vi "AbsoluteIMU-DM.vi"(0 "Operation":u8(ring) items=["Read Accl", "Read Compass", "Read Magnetic Field", "Read Accl & Compass", "Read Gyro", "Begin Compass Calib", "End Compass Calib", "Sens-2G", "Sens-4G", "Sens-8G", "Sens-16G"], 2 "NXT":T3={"Hardware"="NXT", "Flattened String"=""}, 3 "Input Port":T2=3 items=["Port 1", "Port 2", "Port 3", "Port 4"]) -> (1 "output cluster":T1={"X Tilt"=0, "Y Tilt"=0, "Z Tilt"=0, "X Accel"=0, "Y Accel"=0, "Z accel"=0, "X Gyro"=0, "Y Gyro"=0, "Z Gyro"=0, "X Mag"=0, "Y Mag"=0, "Z Mag"=0, "Heading"=0, "Success?"=TRUE}, 4 "NXT dup":T3 caption="NXT")   [LabVIEW 2011]
uses:
  <vilib>/NXT/Subs/LVHSConnector.ctl
  <vilib>/NXT/Block Support/NXT_InputPort.ctl
  <vilib>/NXT/Block Support/HWPage.SensorType.ctl
  <vilib>/NXT/Block Support/HWPage.SensorMode.ctl
panel:
  out "last Z Magnetic Field":i16
  out "last Y Magnetic Field":i16
  out "last X Magnetic Field":i16
  out "Heading":i16
  out "Z Accel":i16
  out "Y Accel":i16
  out "X Accel":i16
  out "Z Tilt":i16
  out "Y Tilt":i16
  out "X Tilt":i16
  out "last Z Gyro":i16
  out "last Y Gyro":i16
  out "last X Gyro":i16
  out "last X Tilt":i16
  out "last Y Tilt":i16
  out "last Z Tilt":i16
  out "last Y Accel":i16
  out "last X Accel":i16
  out "last Z Accel":i16
  out "last Heading":i16
  in  "Address":u8=34 format="%x"
  out "Boolean":bool=TRUE caption="Yes / No"
  out "Y Gyro":i16
  out "X Gyro":i16
  out "Z Gyro":i16
  out "Y Magnetic Field":i16
  out "X Magnetic Field":i16
  out "Z Magnetic Field":i16
  # "mindsensors.com\nCopyright (c) 2013 by mindsensors.com\nEmail: info (<at>) mindsensors (<dot>) com\n\nThis program is free software. You can redistribute it and/or modify\nit under the terms of the GNU General Public License as published by\nthe Free Software Foundation; version 3 of the License.\nRead the license at: http://www.gnu.org/licenses/gpl.txt"
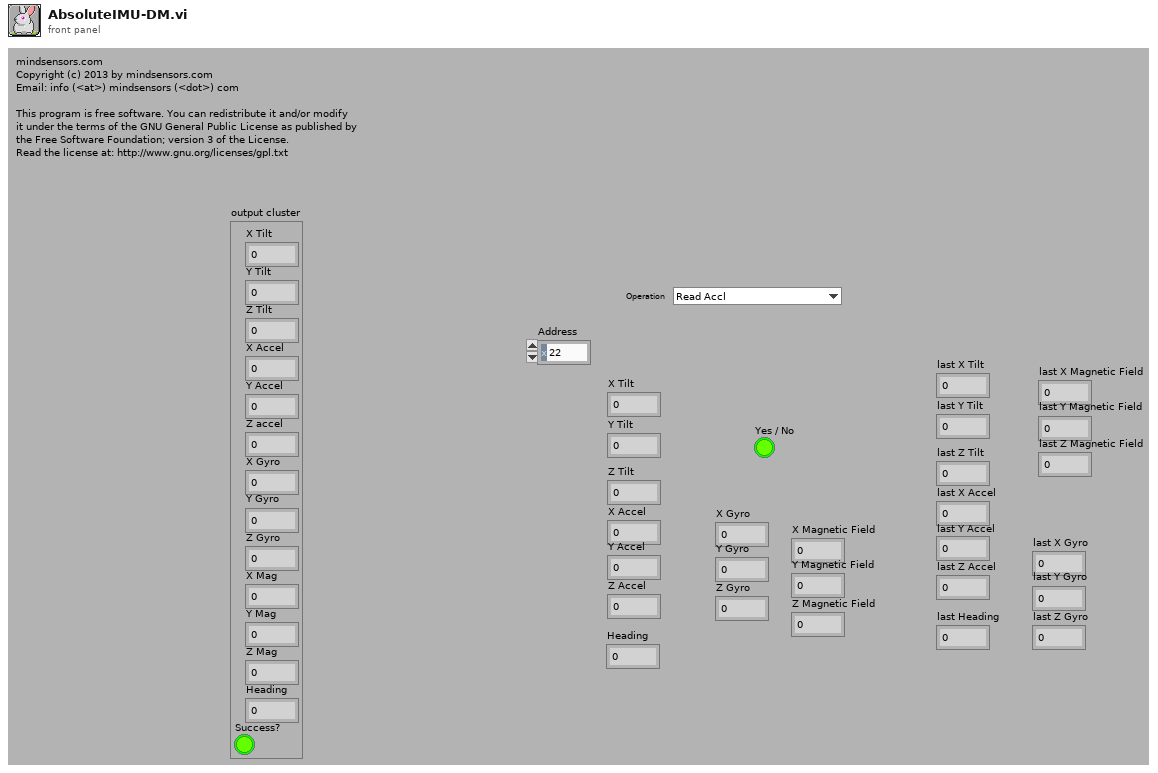
[diagram p1: front panel]
types:
  T1 = cluster{"X Tilt":i32, "Y Tilt":i32, "Z Tilt":i32, "X Accel":i32, "Y Accel":i32, "Z accel":i32, "X Gyro":i32, "Y Gyro":i32, "Z Gyro":i32, "X Mag":i32, "Y Mag":i32, "Z Mag":i32, "Heading":i32, "Success?":bool}
  T2 = typedef "NXT_InputPort.ctl" = u8
  T3 = typedef "LVHSConnector.ctl" = cluster{"Hardware":string, "Flattened String":string}
  T4 = typedef "HWPage.SensorType.ctl" = u8
  T5 = typedef "HWPage.SensorMode.ctl" = u8
  T6 = cluster{i16, i16, i16, i16, i16, i16, i16, i16, i16, i16, i16, i16, "last X Tilt":i32, "Success?":bool}
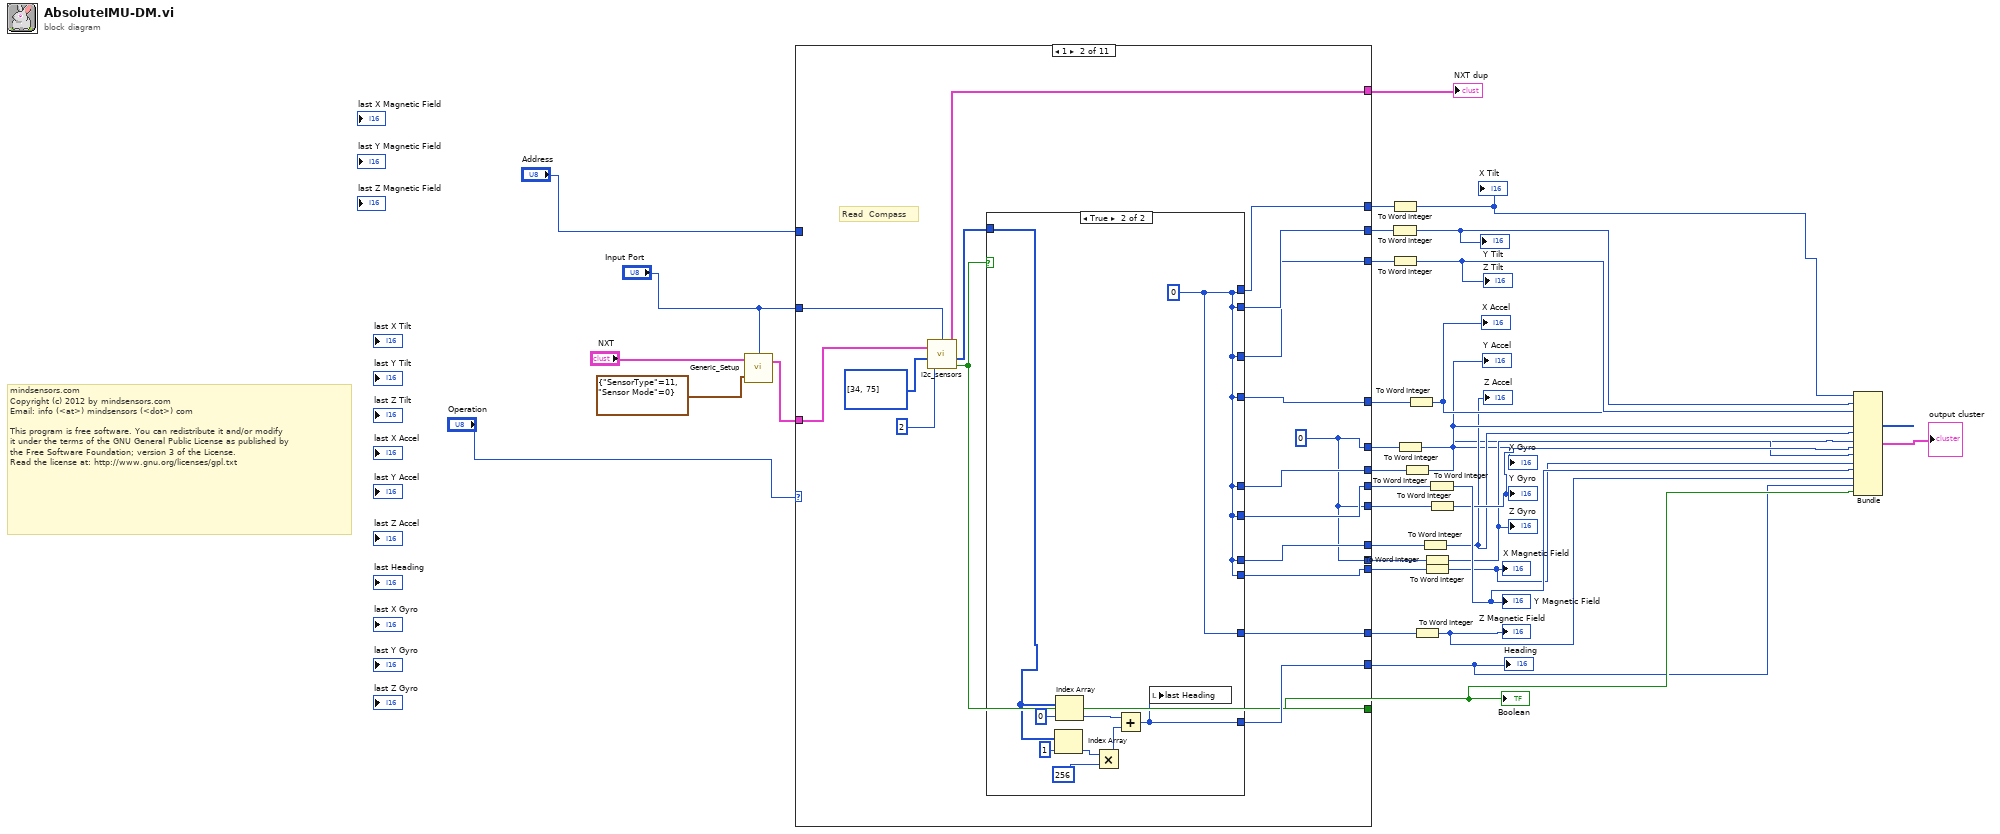
[diagram p0: block diagram]
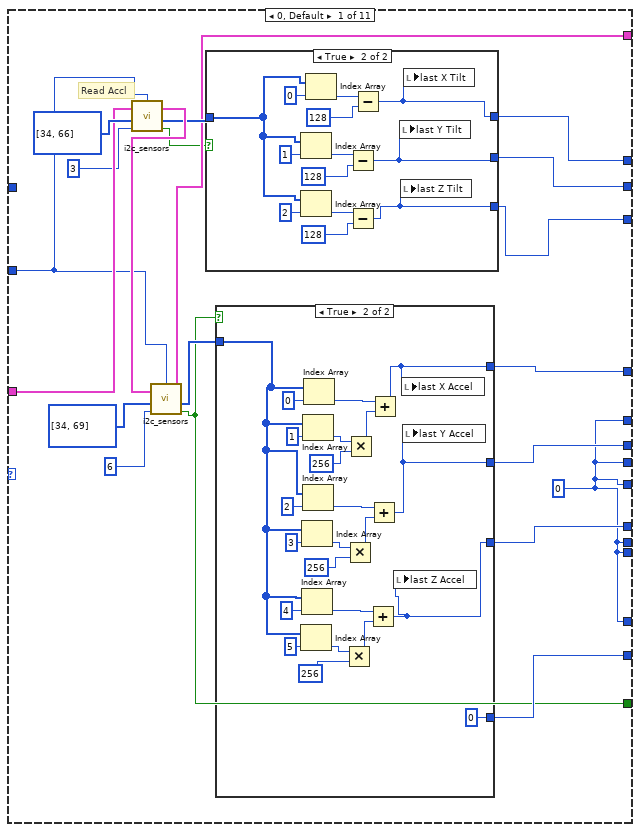
[diagram p2: hidden frame]
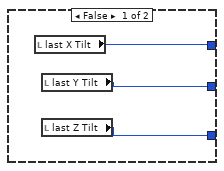
[diagram p3: hidden frame]
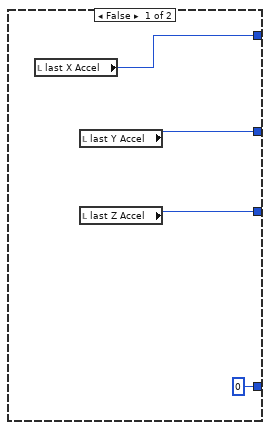
[diagram p4: hidden frame]
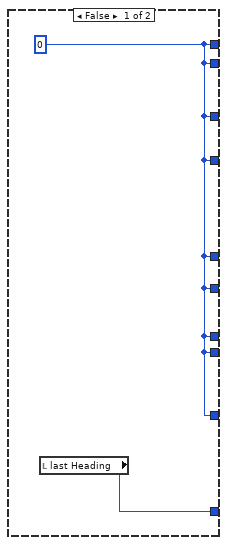
[diagram p5: hidden frame]
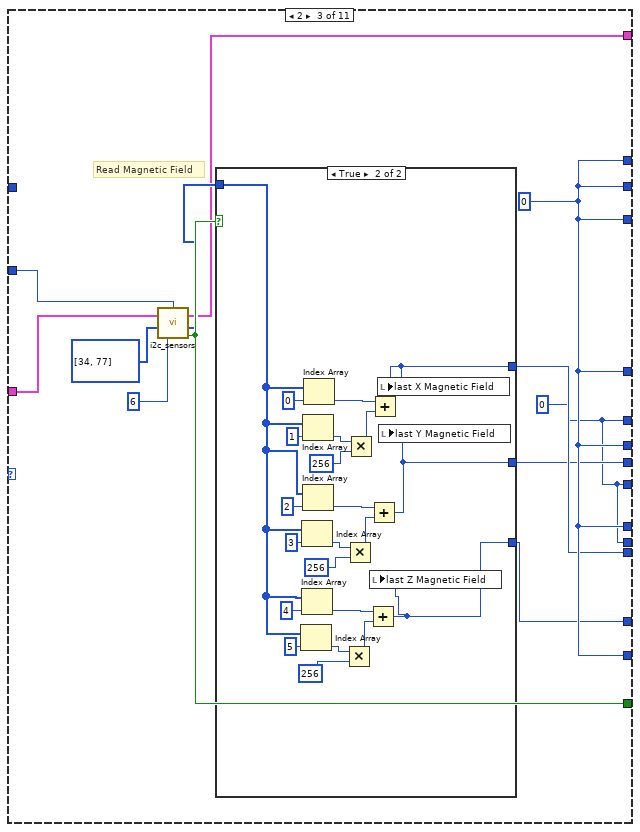
[diagram p6: hidden frame]
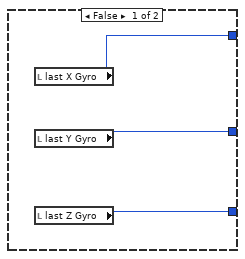
[diagram p7: hidden frame]
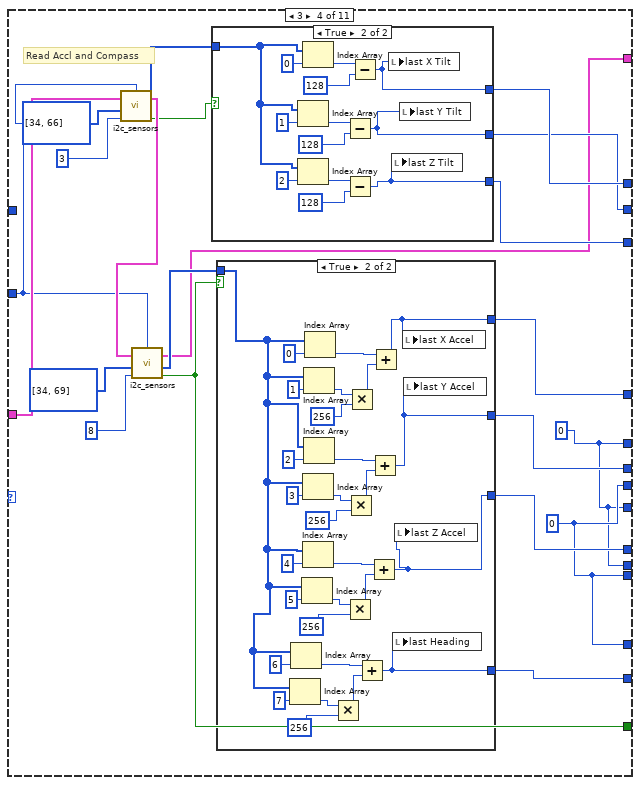
[diagram p8: hidden frame]
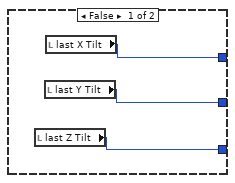
[diagram p9: hidden frame]
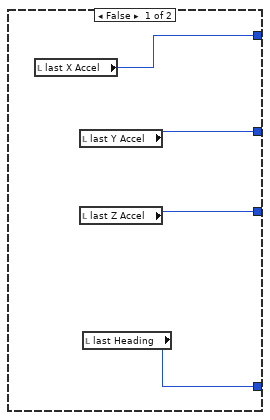
[diagram p10: hidden frame]
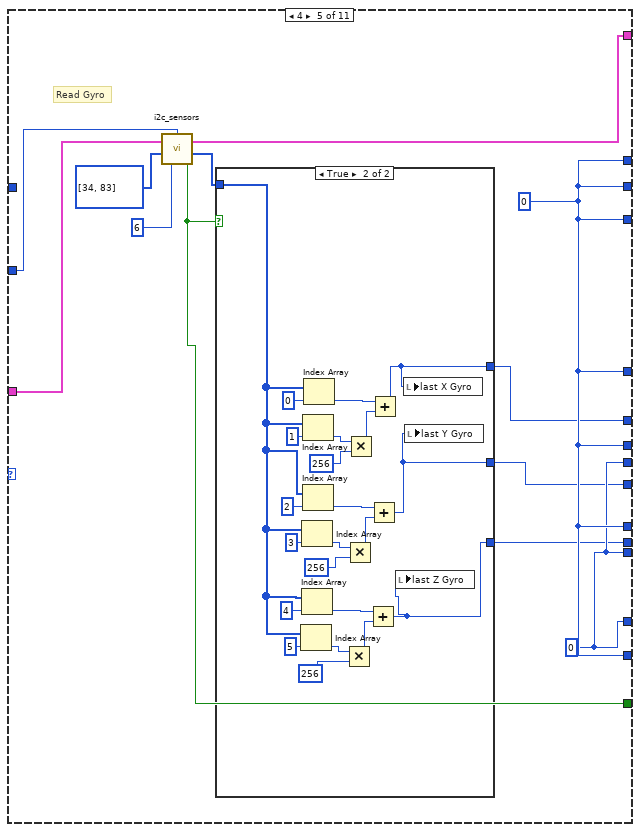
[diagram p11: hidden frame]
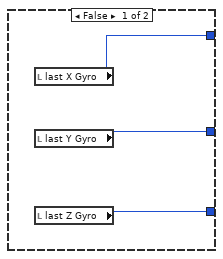
[diagram p12: hidden frame]
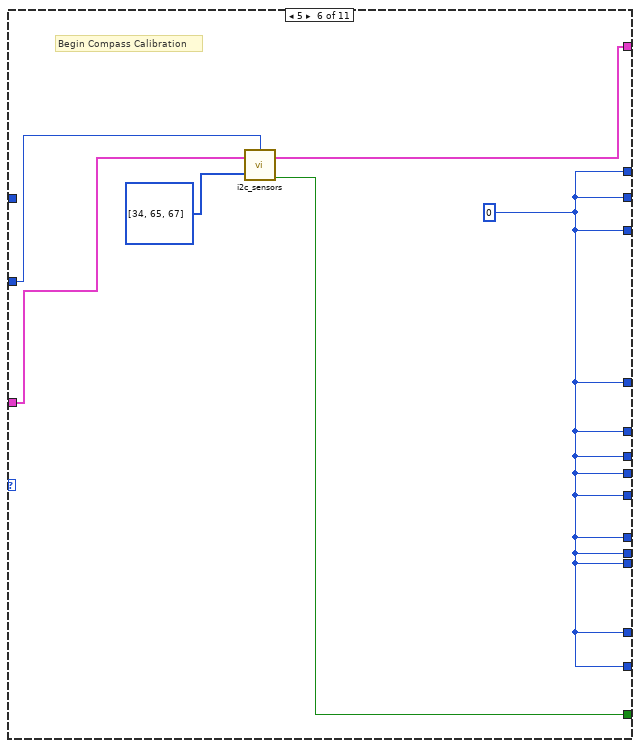
[diagram p13: hidden frame]
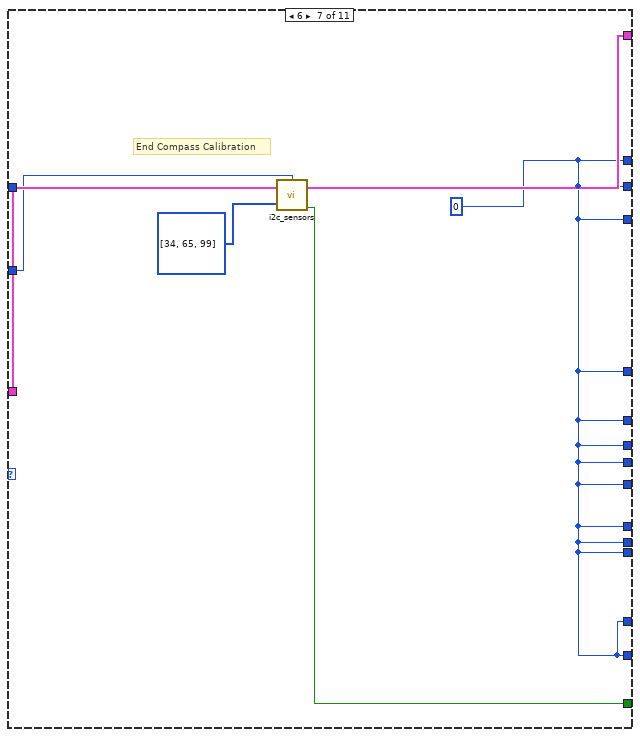
[diagram p14: hidden frame]
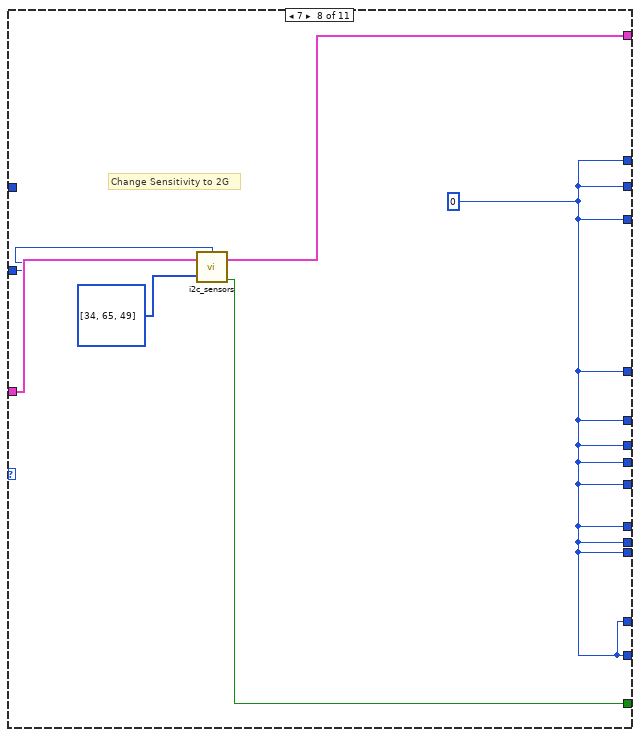
[diagram p15: hidden frame]
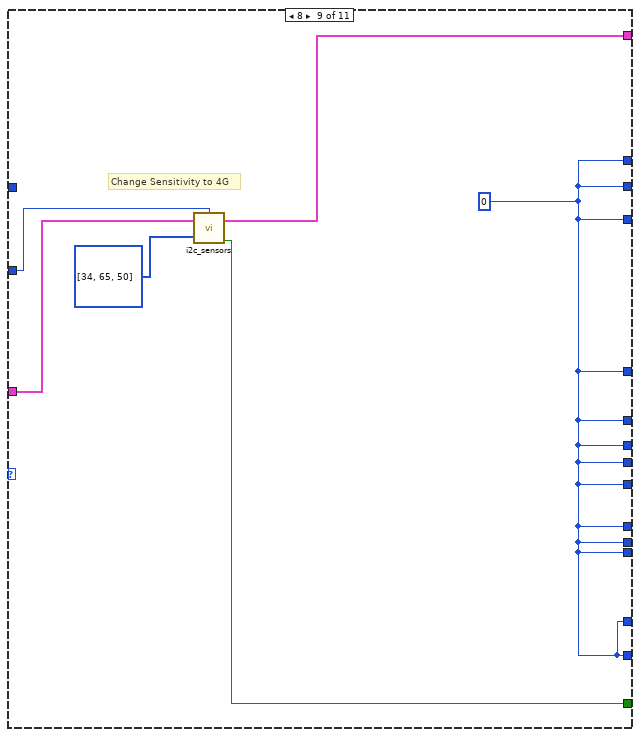
[diagram p16: hidden frame]
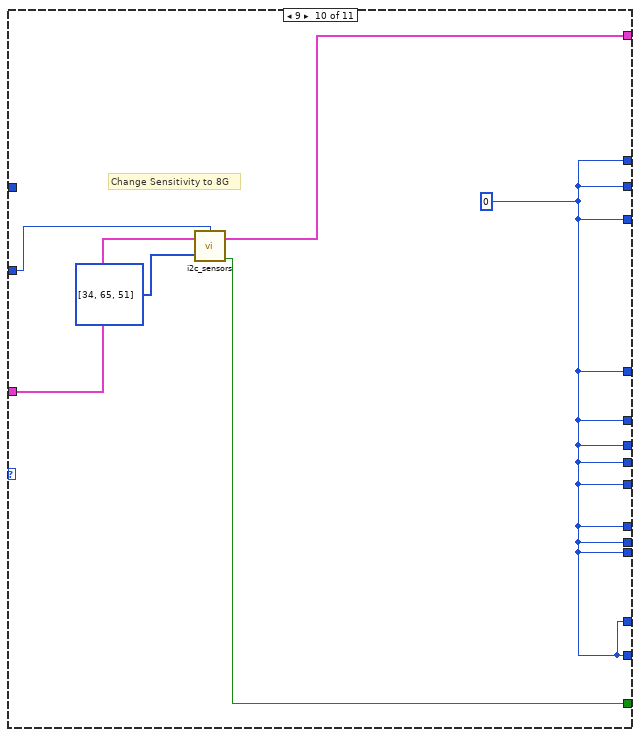
[diagram p17: hidden frame]
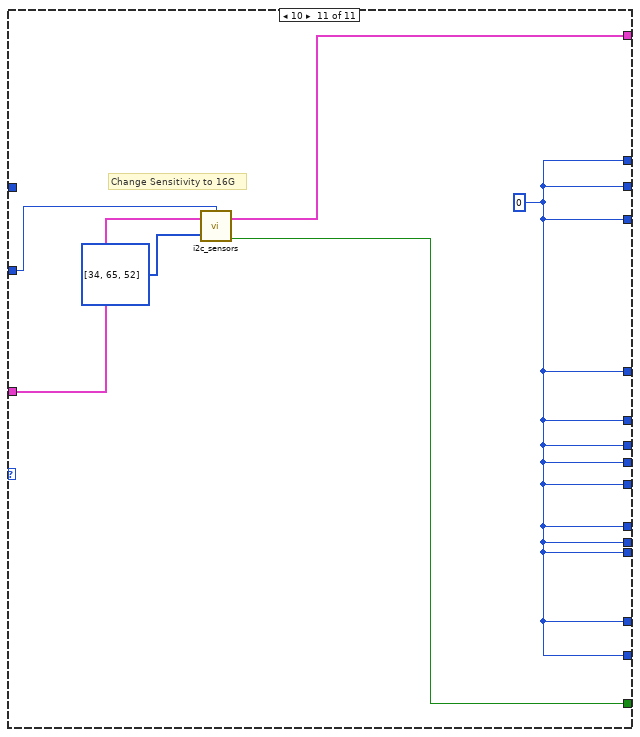
[diagram p18: hidden frame]
diagram:
  # "mindsensors.com\nCopyright (c) 2012 by mindsensors.com\nEmail: info (<at>) mindsensors (<dot>) com\n\nThis program is free software. You can redistribute it and/or modify\nit under the terms of the GNU General Public License as published by\nthe Free Software Foundation; version 3 of the License.\nRead the license at: http://www.gnu.org/licenses/gpl.txt"
  n1 = call <vilib>:"Generic_Setup.vi"("Sensor Setup"=cluster{"SensorType":T4, "Sensor Mode":T5} {"SensorType"=11, "Sensor Mode"=0}, "NXT"="NXT", "Port"="Input Port") -> ("NXT"=w31:T3)  [unwired: 1 out]
  n2 = case shown="1" "Operation" {
    tunnel: "Address" -> [_ _ _ _ _ _ _ _ _ _ _]
    tunnel: [w35 w106 w135 w169 w239 w273 w279 w285 w291 w299 w303] -> w16
    tunnel: [w50 w115 w138 w180 w245 w271 w277 w283 w289 w295 w301] -> w14
    tunnel: [w49 w114 w138 w179 w245 w271 w277 w283 w289 w295 w301] -> w27
    tunnel: [w48 w113 w138 w178 w245 w271 w277 w283 w289 w295 w301] -> w26
    tunnel: [w54 w112 w138 w184 w245 w271 w277 w283 w289 w295 w301] -> w25
    tunnel: [w53 w111 w138 w183 w245 w271 w277 w283 w289 w295 w301] -> w24
    tunnel: [w52 w110 w138 w182 w245 w271 w277 w283 w289 w295 w301] -> w23
    tunnel: [w51 w109 w138 w181 w245 w271 w277 w283 w289 w295 w301] -> w2
    tunnel: w31 -> [w43 w105 w133 w172 w242 w275 w281 w287 w293 w298 w305]
    tunnel: "Input Port" -> [w39 w103 w134 w171 w241 w276 w280 w286 w292 w297 w304]
    tunnel: [w38 w102 w131 w166 w238 w272 w278 w284 w290 w296 w302] -> w30
    tunnel: [w37 w100 w130 w165 w237 w271 w277 w283 w289 w295 w301] -> w19
    tunnel: [w37 w101 w129 w165 w237 w271 w277 w283 w289 w295 w301] -> w18
    tunnel: [w37 w99 w128 w165 w237 w271 w277 w283 w289 w295 w301] -> w17
    tunnel: [w37 w98 w127 w164 w236 w271 w277 w283 w289 w295 w301] -> w22
    tunnel: [w37 w98 w127 w164 w235 w271 w277 w283 w289 w295 w301] -> w21
    tunnel: [w37 w98 w127 w164 w234 w271 w277 w283 w289 w295 w301] -> w20
    frame 0, Default {
      w37 = i16 0 ("last X Tilt")
      # "Read Accl"
      n3 = call <vilib>:"i2c_sensors.vi"("Return Length"=u8 3, "Bytes to Write"=u8[] [34, 66] ("Parameters"), "NXT"=w43, "Port"=w39) -> ("Success?"=w36:bool, "Bytes read"=w40:u8[], "NXT"=w42:T3)  [unwired: 1 in]
      n4 = call <vilib>:"i2c_sensors.vi"("Return Length"=u8 6, "Bytes to Write"=u8[] [34, 69] ("Parameters"), "NXT"=w42, "Port"=w39) -> ("Success?"=w35:bool, "Bytes read"=w45:u8[], "NXT"=w38:T3)  [unwired: 1 in]
      n5 = case shown="True" w36 {
        tunnel: w40 -> [_ w62]
        tunnel: [w55 w61] -> w50
        tunnel: [w57 w60] -> w49
        tunnel: [w56 w59] -> w48
        frame False {
          n6 = local read "last X Tilt"() -> (w55:i16)
          n7 = local read "last Y Tilt"() -> (w57:i16)
          n8 = local read "last Z Tilt"() -> (w56:i16)
        }
        frame True {
          n9 = Index Array(array=w62, index=1) -> (element=w66:u8)
          n10 = Index Array(array=w62, index=2) -> (element=w63:u8)
          n11 = Index Array(array=w62, index=0) -> (element=w58:u8)
          n12 = Subtract(x=w66, y=128) -> (x-y=w60:i32)
          n13 = Subtract(x=w63, y=128) -> (x-y=w59:i32)
          n14 = Subtract(x=w58, y=128) -> (x-y=w61:i32)
          n15 = local write "last Y Tilt"(w60) -> ()
          n16 = local write "last Z Tilt"(w59) -> ()
          n17 = local write "last X Tilt"(w61) -> ()
        }
      }
      n18 = case shown="True" w35 {
        tunnel: w45 -> [_ w75]
        tunnel: [w74 w77] -> w54
        tunnel: [w73 w78] -> w53
        tunnel: [w72 w79] -> w52
        tunnel: [i16 0 ("last Heading") i16 0 ("last Heading")] -> w51
        frame False {
          n19 = local read "last X Accel"() -> (w74:i16)
          n20 = local read "last Y Accel"() -> (w73:i16)
          n21 = local read "last Z Accel"() -> (w72:i16)
        }
        frame True {
          n22 = Index Array(array=w75, index=5) -> (element=w83:u8)
          n23 = Index Array(array=w75, index=3) -> (element=w88:u8)
          n24 = Index Array(array=w75, index=4) -> (element=w85:u8)
          n25 = Index Array(array=w75, index=1) -> (element=w93:u8)
          n26 = Index Array(array=w75, index=2) -> (element=w90:u8)
          n27 = Index Array(array=w75, index=0) -> (element=w95:u8)
          n28 = Multiply(x=w83, y=256) -> (x*y=w84:i32)
          n29 = Multiply(x=w88, y=256) -> (x*y=w89:i32)
          n30 = Multiply(x=w93, y=256) -> (x*y=w94:i32)
          n31 = Add(x=w85, y=w84) -> (x+y=w79:i32)
          n32 = Add(x=w90, y=w89) -> (x+y=w78:i32)
          n33 = Add(x=w95, y=w94) -> (x+y=w77:i32)
          n34 = local write "last Z Accel"(w79) -> ()
          n35 = local write "last X Accel"(w77) -> ()
          n36 = local write "last Y Accel"(w78) -> ()
        }
      }
    }
    frame 1 {
      w98 = i16 0 ("last X Tilt")
      # "Read  Compass"
      n37 = call <vilib>:"i2c_sensors.vi"("Return Length"=u8 2, "Bytes to Write"=u8[] [34, 75] ("Parameters"), "NXT"=w105, "Port"=w103) -> ("Success?"=w106:bool, "Bytes read"=w104:u8[], "NXT"=w102:T3)  [unwired: 1 in]
      n38 = case shown="True" w106 {
        tunnel: [w116 w118] -> w115
        tunnel: w104 -> [_ w120]
        tunnel: [w116 w118] -> w114
        tunnel: [w116 w118] -> w113
        tunnel: [w116 w118] -> w112
        tunnel: [w116 w118] -> w111
        tunnel: [w116 w118] -> w110
        tunnel: [w117 w119] -> w109
        tunnel: [w116 w118] -> w101
        tunnel: [w116 w118] -> w100
        tunnel: [w116 w118] -> w99
        frame False {
          w116 = i16 0 ("last X Tilt")
          n39 = local read "last Heading"() -> (w117:i16)
        }
        frame True {
          w118 = i16 0 ("last X Tilt")
          n40 = Index Array(array=w120, index=1) -> (element=w122:u8)
          n41 = Index Array(array=w120, index=0) -> (element=w124:u8)
          n42 = Multiply(x=w122, y=256) -> (x*y=w123:i32)
          n43 = Add(x=w124, y=w123) -> (x+y=w119:i32)
          n44 = local write "last Heading"(w119) -> ()
        }
      }
    }
    frame 2 {
      w127 = i16 0 ("last X Tilt")
      w138 = 0 ("last X Tilt")
      # "Read Magnetic Field"
      n45 = call <vilib>:"i2c_sensors.vi"("Return Length"=u8 6, "Bytes to Write"=u8[] [34, 77] ("Parameters"), "NXT"=w133, "Port"=w134) -> ("Success?"=w135:bool, "Bytes read"=w132:u8[], "NXT"=w131:T3)  [unwired: 1 in]
      n46 = case shown="True" w135 {
        tunnel: w132 -> [_ w145]
        tunnel: [w141 w142] -> w130
        tunnel: [w140 w143] -> w129
        tunnel: [w139 w144] -> w128
        frame False {
          n47 = local read "last X Gyro"() -> (w141:i16)
          n48 = local read "last Y Gyro"() -> (w140:i16)
          n49 = local read "last Z Gyro"() -> (w139:i16)
        }
        frame True {
          n50 = Index Array(array=w145, index=5) -> (element=w149:u8)
          n51 = Index Array(array=w145, index=3) -> (element=w154:u8)
          n52 = Index Array(array=w145, index=4) -> (element=w151:u8)
          n53 = Index Array(array=w145, index=1) -> (element=w159:u8)
          n54 = Index Array(array=w145, index=2) -> (element=w156:u8)
          n55 = Index Array(array=w145, index=0) -> (element=w161:u8)
          n56 = Multiply(x=w149, y=256) -> (x*y=w150:i32)
          n57 = Multiply(x=w154, y=256) -> (x*y=w155:i32)
          n58 = Multiply(x=w159, y=256) -> (x*y=w160:i32)
          n59 = Add(x=w151, y=w150) -> (x+y=w144:i32)
          n60 = Add(x=w156, y=w155) -> (x+y=w143:i32)
          n61 = Add(x=w161, y=w160) -> (x+y=w142:i32)
          n62 = local write "last Z Magnetic Field"(w144) -> ()
          n63 = local write "last X Magnetic Field"(w142) -> ()
          n64 = local write "last Y Magnetic Field"(w143) -> ()
        }
      }
    }
    frame 3 {
      w164 = i16 0 ("last X Tilt")
      w165 = 0 ("last X Tilt")
      # "Read Accl and Compass"
      n65 = call <vilib>:"i2c_sensors.vi"("Return Length"=u8 3, "Bytes to Write"=u8[] [34, 66] ("Parameters"), "NXT"=w172, "Port"=w171) -> ("Success?"=w170:bool, "Bytes read"=w167:u8[], "NXT"=w174:T3)  [unwired: 1 in]
      n66 = call <vilib>:"i2c_sensors.vi"("Return Length"=u8 8, "Bytes to Write"=u8[] [34, 69] ("Parameters"), "NXT"=w174, "Port"=w171) -> ("Success?"=w169:bool, "Bytes read"=w168:u8[], "NXT"=w166:T3)  [unwired: 1 in]
      n67 = case shown="True" w170 {
        tunnel: w167 -> [_ w191]
        tunnel: [w187 w190] -> w180
        tunnel: [w186 w189] -> w179
        tunnel: [w185 w188] -> w178
        frame False {
          n68 = local read "last Z Tilt"() -> (w185:i16)
          n69 = local read "last Y Tilt"() -> (w186:i16)
          n70 = local read "last X Tilt"() -> (w187:i16)
        }
        frame True {
          n71 = Index Array(array=w191, index=1) -> (element=w197:u8)
          n72 = Index Array(array=w191, index=2) -> (element=w200:u8)
          n73 = Index Array(array=w191, index=0) -> (element=w193:u8)
          n74 = Subtract(x=w197, y=128) -> (x-y=w189:i32)
          n75 = Subtract(x=w200, y=128) -> (x-y=w188:i32)
          n76 = Subtract(x=w193, y=128) -> (x-y=w190:i32)
          n77 = local write "last X Tilt"(w190) -> ()
          n78 = local write "last Z Tilt"(w188) -> ()
          n79 = local write "last Y Tilt"(w189) -> ()
        }
      }
      n80 = case shown="True" w169 {
        tunnel: w168 -> [_ w205]
        tunnel: [w204 w206] -> w184
        tunnel: [w203 w207] -> w183
        tunnel: [w202 w208] -> w182
        tunnel: [w201 w209] -> w181
        frame False {
          n81 = local read "last X Accel"() -> (w204:i16)
          n82 = local read "last Y Accel"() -> (w203:i16)
          n83 = local read "last Z Accel"() -> (w202:i16)
          n84 = local read "last Heading"() -> (w201:i16)
        }
        frame True {
          n85 = Index Array(array=w205, index=7) -> (element=w211:u8)
          n86 = Index Array(array=w205, index=6) -> (element=w213:u8)
          n87 = Index Array(array=w205, index=5) -> (element=w219:u8)
          n88 = Index Array(array=w205, index=3) -> (element=w224:u8)
          n89 = Index Array(array=w205, index=4) -> (element=w221:u8)
          n90 = Index Array(array=w205, index=1) -> (element=w229:u8)
          n91 = Index Array(array=w205, index=2) -> (element=w226:u8)
          n92 = Index Array(array=w205, index=0) -> (element=w231:u8)
          n93 = Multiply(x=w211, y=256) -> (x*y=w212:i32)
          n94 = Multiply(x=w219, y=256) -> (x*y=w220:i32)
          n95 = Multiply(x=w224, y=256) -> (x*y=w225:i32)
          n96 = Multiply(x=w229, y=256) -> (x*y=w230:i32)
          n97 = Add(x=w213, y=w212) -> (x+y=w209:i32)
          n98 = Add(x=w221, y=w220) -> (x+y=w208:i32)
          n99 = Add(x=w226, y=w225) -> (x+y=w207:i32)
          n100 = Add(x=w231, y=w230) -> (x+y=w206:i32)
          n101 = local write "last Heading"(w209) -> ()
          n102 = local write "last Z Accel"(w208) -> ()
          n103 = local write "last X Accel"(w206) -> ()
          n104 = local write "last Y Accel"(w207) -> ()
        }
      }
    }
    frame 4 {
      w237 = 0 ("last X Tilt")
      w245 = 0 ("last X Tilt")
      # "Read Gyro"
      n105 = call <vilib>:"i2c_sensors.vi"("Return Length"=u8 6, "Bytes to Write"=u8[] [34, 83] ("Parameters"), "NXT"=w242, "Port"=w241) -> ("Success?"=w239:bool, "Bytes read"=w240:u8[], "NXT"=w238:T3)  [unwired: 1 in]
      n106 = case shown="True" w239 {
        tunnel: w240 -> [_ w252]
        tunnel: [w248 w249] -> w236
        tunnel: [w247 w250] -> w235
        tunnel: [w246 w251] -> w234
        frame False {
          n107 = local read "last X Gyro"() -> (w248:i16)
          n108 = local read "last Y Gyro"() -> (w247:i16)
          n109 = local read "last Z Gyro"() -> (w246:i16)
        }
        frame True {
          n110 = Index Array(array=w252, index=5) -> (element=w256:u8)
          n111 = Index Array(array=w252, index=3) -> (element=w261:u8)
          n112 = Index Array(array=w252, index=4) -> (element=w258:u8)
          n113 = Index Array(array=w252, index=1) -> (element=w266:u8)
          n114 = Index Array(array=w252, index=2) -> (element=w263:u8)
          n115 = Index Array(array=w252, index=0) -> (element=w268:u8)
          n116 = Multiply(x=w256, y=256) -> (x*y=w257:i32)
          n117 = Multiply(x=w261, y=256) -> (x*y=w262:i32)
          n118 = Multiply(x=w266, y=256) -> (x*y=w267:i32)
          n119 = Add(x=w258, y=w257) -> (x+y=w251:i32)
          n120 = Add(x=w263, y=w262) -> (x+y=w250:i32)
          n121 = Add(x=w268, y=w267) -> (x+y=w249:i32)
          n122 = local write "last Z Gyro"(w251) -> ()
          n123 = local write "last X Gyro"(w249) -> ()
          n124 = local write "last Y Gyro"(w250) -> ()
        }
      }
    }
    frame 5 {
      w271 = 0 ("last X Tilt")
      # "Begin Compass Calibration"
      n125 = call <vilib>:"i2c_sensors.vi"("Bytes to Write"=u8[] [34, 65, 67] ("Parameters"), "NXT"=w275, "Port"=w276) -> ("Success?"=w273:bool, "NXT"=w272:T3)  [unwired: 2 in, 1 out]
    }
    frame 6 {
      w277 = 0 ("last X Tilt")
      # "End Compass Calibration"
      n126 = call <vilib>:"i2c_sensors.vi"("Bytes to Write"=u8[] [34, 65, 99] ("Parameters"), "NXT"=w281, "Port"=w280) -> ("Success?"=w279:bool, "NXT"=w278:T3)  [unwired: 2 in, 1 out]
    }
    frame 7 {
      w283 = 0 ("last X Tilt")
      # "Change Sensitivity to 2G"
      n127 = call <vilib>:"i2c_sensors.vi"("Bytes to Write"=u8[] [34, 65, 49] ("Parameters"), "NXT"=w287, "Port"=w286) -> ("Success?"=w285:bool, "NXT"=w284:T3)  [unwired: 2 in, 1 out]
    }
    frame 8 {
      w289 = 0 ("last X Tilt")
      # "Change Sensitivity to 4G"
      n128 = call <vilib>:"i2c_sensors.vi"("Bytes to Write"=u8[] [34, 65, 50] ("Parameters"), "NXT"=w293, "Port"=w292) -> ("Success?"=w291:bool, "NXT"=w290:T3)  [unwired: 2 in, 1 out]
    }
    frame 9 {
      w295 = 0 ("last X Tilt")
      # "Change Sensitivity to 8G"
      n129 = call <vilib>:"i2c_sensors.vi"("Bytes to Write"=u8[] [34, 65, 51] ("Parameters"), "NXT"=w298, "Port"=w297) -> ("Success?"=w299:bool, "NXT"=w296:T3)  [unwired: 2 in, 1 out]
    }
    frame 10 {
      w301 = 0 ("last X Tilt")
      # "Change Sensitivity to 16G"
      n130 = call <vilib>:"i2c_sensors.vi"("Bytes to Write"=u8[] [34, 65, 52] ("Parameters"), "NXT"=w305, "Port"=w304) -> ("Success?"=w303:bool, "NXT"=w302:T3)  [unwired: 2 in, 1 out]
    }
  }
  "NXT dup" <- w30
  "Boolean" <- w16
  "Heading" <- w2
  n131 = To Word Integer(number=w27) -> (16bit integer=w12:i16)
  "Y Tilt" <- w12
  n132 = To Word Integer(number=w14) -> (16bit integer=w13:i16)
  "X Tilt" <- w13
  n133 = To Word Integer(number=w26) -> (16bit integer=w11:i16)
  "Z Tilt" <- w11
  n134 = To Word Integer(number=w22) -> (16bit integer=w1:i16)
  "X Gyro" <- w1
  n135 = To Word Integer(number=w24) -> (16bit integer=w9:i16)
  "Y Accel" <- w9
  n136 = To Word Integer(number=w25) -> (16bit integer=w10:i16)
  "X Accel" <- w10
  n137 = To Word Integer(number=w17) -> (16bit integer=w3:i16)
  "Z Magnetic Field" <- w3
  n138 = To Word Integer(number=w23) -> (16bit integer=w6:i16)
  "Z Accel" <- w6
  n139 = To Word Integer(number=w20) -> (16bit integer=w5:i16)
  "Z Gyro" <- w5
  n140 = To Word Integer(number=w19) -> (16bit integer=w4:i16)
  "X Magnetic Field" <- w4
  n141 = To Word Integer(number=w18) -> (16bit integer=w8:i16)
  "Y Magnetic Field" <- w8
  n142 = To Word Integer(number=w21) -> (16bit integer=w7:i16)
  "Y Gyro" <- w7
  n143 = Bundle(w13, w12, w11, w10, w9, w6, w1, w7, w5, w4, w8, w3, "last X Tilt"=w2, "Success?"=w16) -> (→"output cluster":T6)  [unwired: 1 in]
